vi "SMU_IV dual.vi"() -> ()   [LabVIEW 2022 SP3]
uses:
  <vilib>/Analysis/1siggen.llb/Ramp Pattern by Delta.vi
  Agilent U2722/Public/Configure/Configure Channel (Current).vi
  Agilent U2722/Public/Configure/Configure Channel (Voltage).vi
  Agilent U2722/Public/Data/Read Output (Single).vi
  <vilib>/Utility/file.llb/Write Delimited Spreadsheet (DBL).vi
  Agilent U2722/Agilent U2722.lvlib
  <vilib>/Analysis/NI_AALBase.lvlib
panel:
  in  "Tab Control":enum32{"Device Setup"}(tab)
  in  "Voltage Range 2":u16(ring) items=["2 Volts", "20 Volts"]
  in  "Current Range 2":u16(ring)=4 items=["1 uA", "10 uA", "100 uA", "1 mA", "10 mA", "120 mA"]
  in  "Current Limit  2":dbl=0.005 format="%#_2p"
  in  "Voltage Range":u16(ring) items=["2 Volts", "20 Volts"]
  in  "Starting Voltage (V)":dbl
  in  "Stopping Voltage (V)":dbl=1.0
  in  "Voltage Interval  (DV)":dbl format="%#_2g"
  in  "Current Range":u16(ring)=4 items=["1 uA", "10 uA", "100 uA", "1 mA", "10 mA", "120 mA"]
  in  "VISA resource name":refnum<visa-resource-name>
  in  "Drain - Source Channel":u16(ring)=1 items=["Channel 1"=1, "Channel 2"=2, "Channel 3"=3]
  in  "PLC":i32
  in  "Current Limit":dbl=0.005 format="%#_2p"
  in  "Interval Time (s)":dbl=1.0 caption="Delay Time (s)"
  in  "Starting Voltage (V) 2":dbl
  in  "Stopping Voltage (V) 2":dbl=1.0
  in  "Voltage Interval 2 (DV)":dbl format="%#_2g"
  in  "Gate - Source Channel":u16(ring)=2 items=["Channel 1"=1, "Channel 2"=2, "Channel 3"=3]
  in  "output file path":path
  out "XY Graph":cluster{"Y":dbl[], "Y":dbl[]}[](graph)
  out "XY Graph 2":cluster{"Y":dbl[], "Y":dbl[]}[](graph)
  out "XY Graph 4":cluster{"Y":dbl[], "Y":dbl[]}[](graph)
  out "XY Graph 3":cluster{"Y":dbl[], "Y":dbl[]}[](graph)
  in  "VISA resource name 2":refnum<visa-resource-name>
  in  "Voltage Range 3":u16(ring) items=["2 Volts", "20 Volts"]
  in  "Starting Voltage (V) 3":dbl
  in  "Stopping Voltage (V) 3":dbl=1.0
  in  "Voltage Interval  (DV) 2":dbl format="%#_2g"
  in  "Current Range 3":u16(ring)=4 items=["1 uA", "10 uA", "100 uA", "1 mA", "10 mA", "120 mA"]
  in  "Drain - Source Channel  2":u16(ring)=1 items=["Channel 1"=1, "Channel 2"=2, "Channel 3"=3]
  in  "PLC 2":i32
  in  "Current Limit  4":dbl=0.005 format="%#_2p"
  in  "Interval Time (s) 2":dbl=1.0 caption="Delay Time (s)"
  in  "Starting Voltage (V) 4":dbl
  in  "Stopping Voltage (V) 4":dbl=1.0
  in  "Voltage Interval 2 (DV)\n 2":dbl format="%#_2g"
  in  "Gate - Source Channel  2":u16(ring)=2 items=["Channel 1"=1, "Channel 2"=2, "Channel 3"=3]
  in  "output file path 2":path
  in  "Current Limit  3":dbl=0.005 format="%#_2p"
  in  "Current Range 4":u16(ring)=4 items=["1 uA", "10 uA", "100 uA", "1 mA", "10 mA", "120 mA"]
  in  "Voltage Range 2":u16(ring) items=["2 Volts", "20 Volts"]
  # "Drain Source Voltage Setting"
  # "Gate Source Voltage Setting"
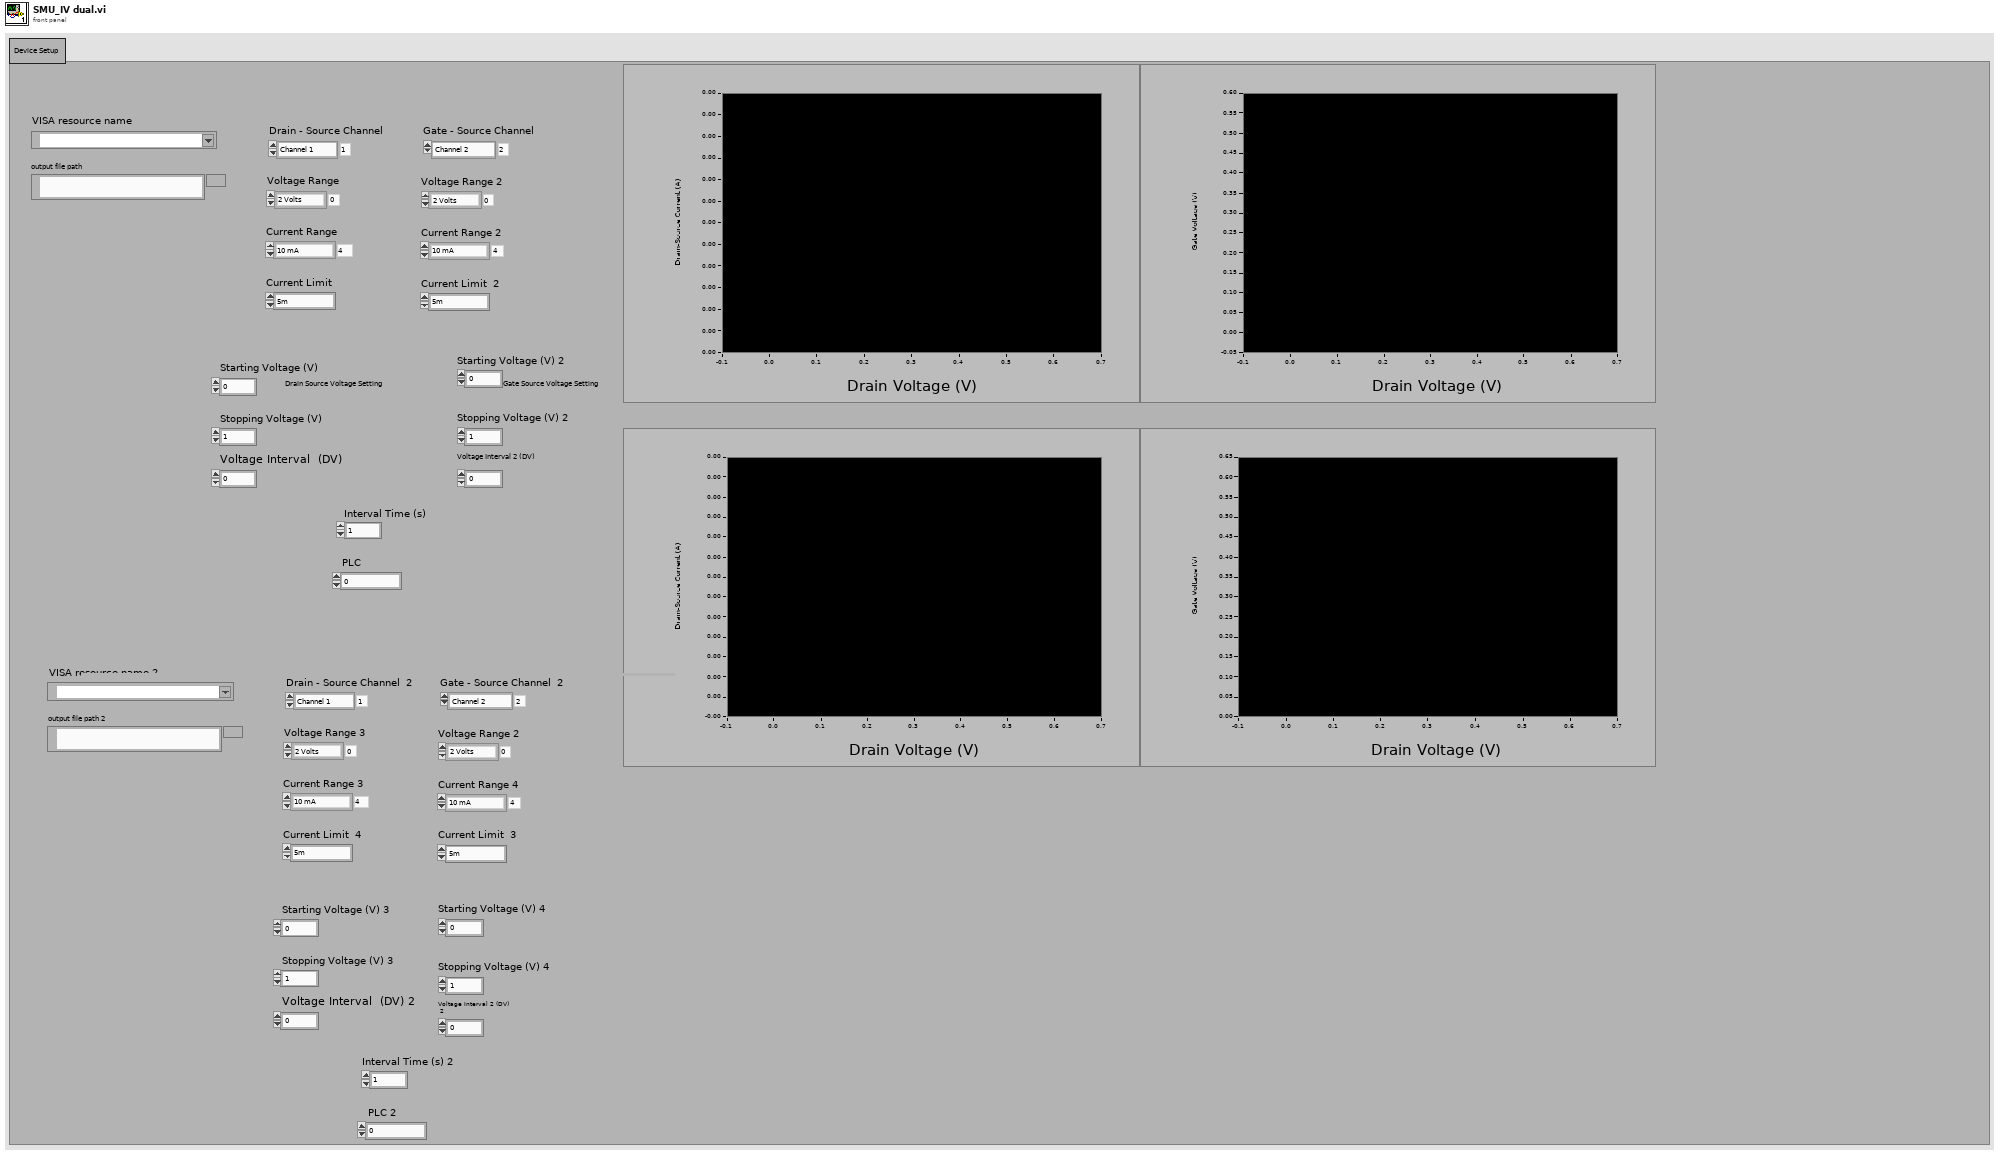
[diagram p1: front panel]
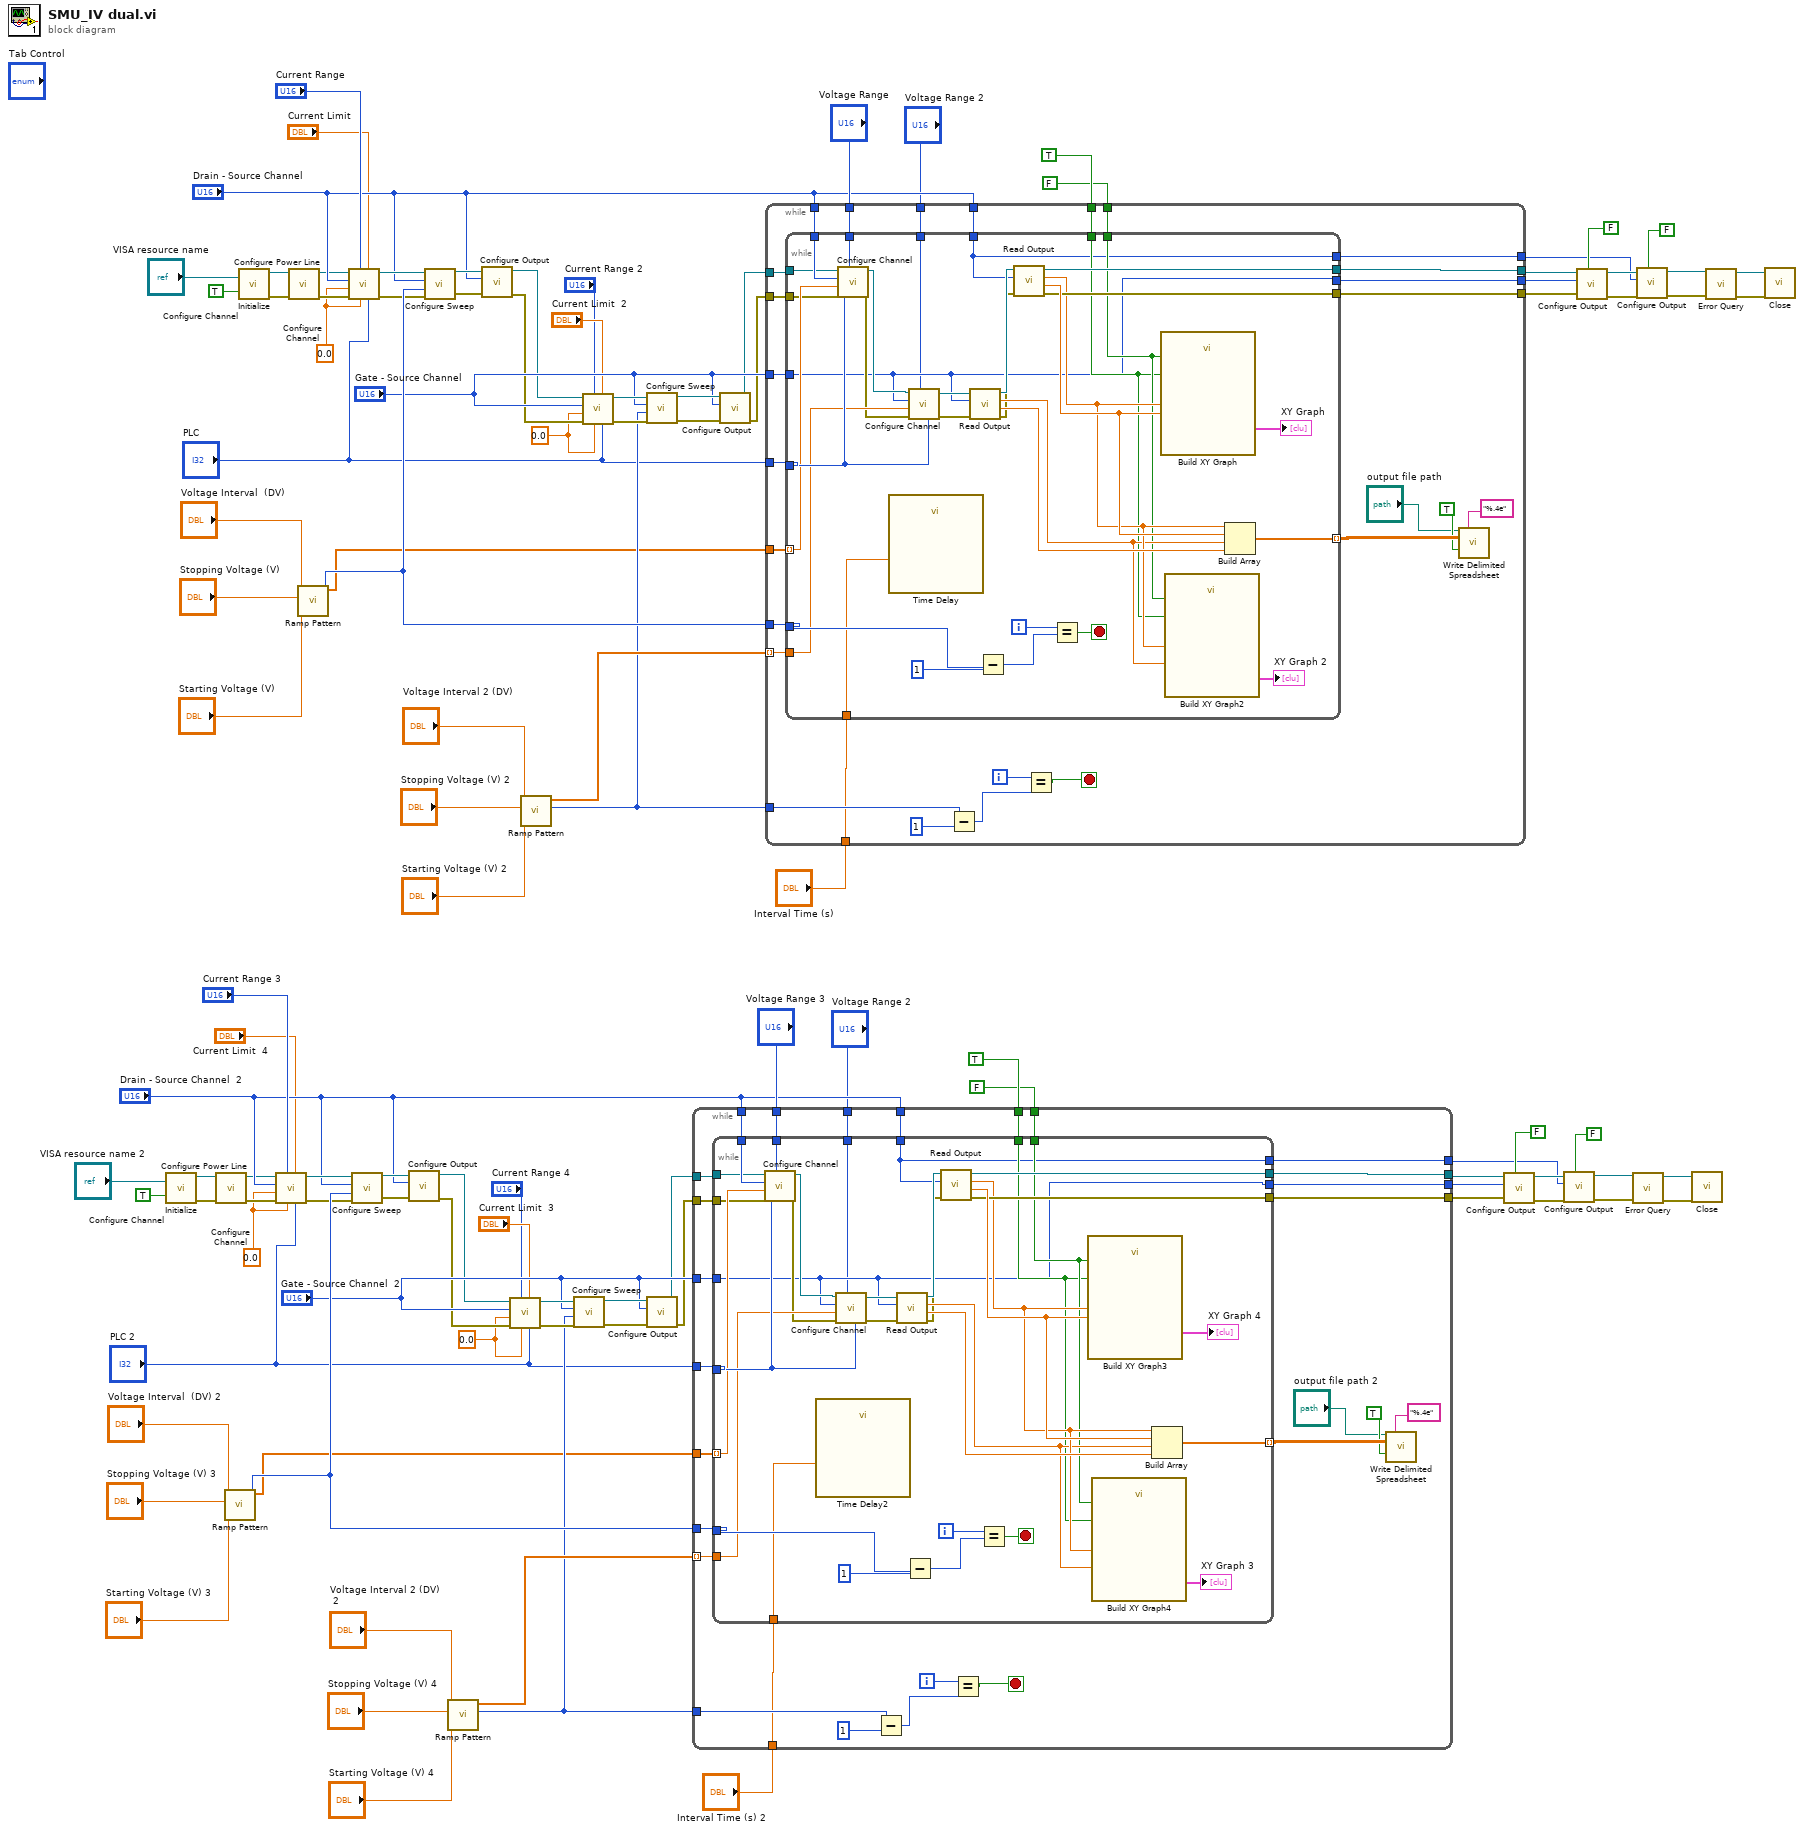
[diagram p0: block diagram]
diagram:
  w3 = 0.0
  w2 = 0.0
  w57 = 0.0
  w56 = 0.0
  n1 = call "Initialize.vi"("ID Query (True)"=TRUE, "VISA resource name"="VISA resource name 2") -> ("error out"=w49:errorcluster, "VISA resource name out"=w48:refnum<visa-resource-name>)  [unwired: 8 in]
  n2 = call "Configure Power Line.vi"("error in (no error)"=w49, "VISA resource name"=w48) -> ("error out"=w32:errorcluster, "VISA resource name out"=w19:refnum<visa-resource-name>)  [unwired: 8 in]
  n3 = call-poly <vilib>:"Ramp Pattern.vi"("start"="Starting Voltage (V) 3", "end"="Stopping Voltage (V) 3", "delta"="Voltage Interval  (DV) 2") -> ("samples"=w39:i32, "Ramp Pattern"=w22:dbl[])  [unwired: 6 in, 1 out]
  n4 = call "Initialize.vi"("ID Query (True)"=TRUE, "VISA resource name"="VISA resource name") -> ("error out"=w103:errorcluster, "VISA resource name out"=w102:refnum<visa-resource-name>)  [unwired: 8 in]
  n5 = call-poly "Configure Channel.vi"("Power Line Cycles (0)"="PLC 2", "Current Limit (1.0 uA)"="Current Limit  4", "Triggered Level (1.0 mA)"=w2, "Current Range (0: 1 uA)"="Current Range 3", "error in (no error)"=w32, "Output Level (1.0 mA)"=w2, "Channel (1: Channel 1)"="Drain - Source Channel  2", "VISA resource name"=w19) -> ("error out"=w36:errorcluster, "VISA resource name out"=w37:refnum<visa-resource-name>)  [unwired: 2 in]
  n6 = call "Configure Power Line.vi"("error in (no error)"=w103, "VISA resource name"=w102) -> ("error out"=w86:errorcluster, "VISA resource name out"=w73:refnum<visa-resource-name>)  [unwired: 8 in]
  n7 = call-poly <vilib>:"Ramp Pattern.vi"("start"="Starting Voltage (V)", "end"="Stopping Voltage (V)", "delta"="Voltage Interval  (DV)") -> ("samples"=w93:i32, "Ramp Pattern"=w76:dbl[])  [unwired: 6 in, 1 out]
  n8 = call-poly "Configure Channel.vi"("Power Line Cycles (0)"="PLC", "Current Limit (1.0 uA)"="Current Limit", "Triggered Level (1.0 mA)"=w56, "Current Range (0: 1 uA)"="Current Range", "error in (no error)"=w86, "Output Level (1.0 mA)"=w56, "Channel (1: Channel 1)"="Drain - Source Channel", "VISA resource name"=w73) -> ("error out"=w90:errorcluster, "VISA resource name out"=w91:refnum<visa-resource-name>)  [unwired: 2 in]
  n9 = call "Configure Sweep.vi"("error in (no error)"=w36, "Sweep Points (1)"=w39, "Channel (1: Channel 1)"="Drain - Source Channel  2", "VISA resource name"=w37) -> ("error out"=w40:errorcluster, "VISA resource name out"=w41:refnum<visa-resource-name>)  [unwired: 6 in]
  n10 = call "Configure Output.vi"("error in (no error)"=w40, "Channel (1: Channel 1)"="Drain - Source Channel  2", "VISA resource name"=w41) -> ("error out"=w17:errorcluster, "VISA resource name out"=w18:refnum<visa-resource-name>)  [unwired: 7 in]
  n11 = call "Configure Sweep.vi"("error in (no error)"=w90, "Sweep Points (1)"=w93, "Channel (1: Channel 1)"="Drain - Source Channel", "VISA resource name"=w91) -> ("error out"=w94:errorcluster, "VISA resource name out"=w95:refnum<visa-resource-name>)  [unwired: 6 in]
  n12 = call-poly <vilib>:"Ramp Pattern.vi"("start"="Starting Voltage (V) 4", "end"="Stopping Voltage (V) 4", "delta"="Voltage Interval 2 (DV)\n 2") -> ("samples"=w25:i32, "Ramp Pattern"=w26:dbl[])  [unwired: 6 in, 1 out]
  n13 = call "Configure Output.vi"("error in (no error)"=w94, "Channel (1: Channel 1)"="Drain - Source Channel", "VISA resource name"=w95) -> ("error out"=w71:errorcluster, "VISA resource name out"=w72:refnum<visa-resource-name>)  [unwired: 7 in]
  n14 = call-poly "Configure Channel.vi"("Power Line Cycles (0)"="PLC 2", "Current Limit (1.0 uA)"="Current Limit  3", "Triggered Level (1.0 mA)"=w3, "Current Range (0: 1 uA)"="Current Range 4", "error in (no error)"=w17, "Output Level (1.0 mA)"=w3, "Channel (1: Channel 1)"="Gate - Source Channel  2", "VISA resource name"=w18) -> ("error out"=w31:errorcluster, "VISA resource name out"=w30:refnum<visa-resource-name>)  [unwired: 2 in]
  n15 = call-poly <vilib>:"Ramp Pattern.vi"("start"="Starting Voltage (V) 2", "end"="Stopping Voltage (V) 2", "delta"="Voltage Interval 2 (DV)") -> ("samples"=w79:i32, "Ramp Pattern"=w80:dbl[])  [unwired: 6 in, 1 out]
  n16 = call "Configure Sweep.vi"("error in (no error)"=w31, "Sweep Points (1)"=w25, "Channel (1: Channel 1)"="Gate - Source Channel  2", "VISA resource name"=w30) -> ("error out"=w28:errorcluster, "VISA resource name out"=w29:refnum<visa-resource-name>)  [unwired: 6 in]
  n17 = call-poly "Configure Channel.vi"("Power Line Cycles (0)"="PLC", "Current Limit (1.0 uA)"="Current Limit  2", "Triggered Level (1.0 mA)"=w57, "Current Range (0: 1 uA)"="Current Range 2", "error in (no error)"=w71, "Output Level (1.0 mA)"=w57, "Channel (1: Channel 1)"="Gate - Source Channel", "VISA resource name"=w72) -> ("error out"=w85:errorcluster, "VISA resource name out"=w84:refnum<visa-resource-name>)  [unwired: 2 in]
  n18 = call "Configure Sweep.vi"("error in (no error)"=w85, "Sweep Points (1)"=w79, "Channel (1: Channel 1)"="Gate - Source Channel", "VISA resource name"=w84) -> ("error out"=w82:errorcluster, "VISA resource name out"=w83:refnum<visa-resource-name>)  [unwired: 6 in]
  n19 = call "Configure Output.vi"("error in (no error)"=w28, "Channel (1: Channel 1)"="Gate - Source Channel  2", "VISA resource name"=w29) -> ("error out"=w16:errorcluster, "VISA resource name out"=w15:refnum<visa-resource-name>)  [unwired: 7 in]
  n20 = while {
    tunnel: TRUE -> [w135]
    tunnel: FALSE -> [w134]
    tunnel: "PLC 2" -> [w133]
    tunnel: "Interval Time (s) 2" -> [w118]
    tunnel: w39 -> [w132]
    tunnel: "Voltage Range 3" -> [w131]
    tunnel: "Gate - Source Channel  2" -> [w130]
    tunnel: w26 -> [w129] mode=indexing
    tunnel: w25 -> [w125]
    tunnel: [w123] -> w24
    tunnel: [w122] -> w23
    tunnel: w22 -> [w121]
    tunnel: "Drain - Source Channel  2" -> [w120]
    tunnel: "Drain - Source Channel  2" -> [w119]
    tunnel: w16 -> [w110]
    tunnel: w15 -> [w117]
    tunnel: [w112] -> w9
    tunnel: [w111] -> w8
    tunnel: "Voltage Range 2" -> [w109]
    i -> [w127]
    stop <- w126 stop-if-true
    n21 = while {
      tunnel: w132 -> [w165]
      tunnel: w118 -> [w164]
      tunnel: w133 -> [w160]
      tunnel: w135 -> [w141]
      tunnel: w134 -> [w142]
      tunnel: [w149] -> w123
      tunnel: [w162] -> w122
      tunnel: w130 -> [w140]
      tunnel: w131 -> [w137]
      tunnel: w129 -> [w159]
      tunnel: [w152] -> w115 mode=indexing
      tunnel: w121 -> [w151] mode=indexing
      tunnel: w120 -> [w150]
      tunnel: w119 -> [w139]
      tunnel: w117 -> [w146]
      tunnel: [w140] -> w112
      tunnel: [w139] -> w111
      tunnel: w110 -> [w138]
      tunnel: w109 -> [w136]
      i -> [w161]
      stop <- w163 stop-if-true
      n22 = call-poly "Configure Channel.vi"("Power Line Cycles (0)"=w160, "Voltage Range (0: 2 Volts)"=w137, "error in (no error)"=w138, "Output Level (1.0 V)"=w151, "Channel (1: Channel 1)"=w150, "VISA resource name"=w146) -> ("error out"=w144:errorcluster, "VISA resource name out"=w145:refnum<visa-resource-name>)  [unwired: 4 in]
      n23 = call "Time Delay2"("Delay Time (s)"=w164) -> ()  [unwired: 10 in, 1 out]
      n24 = call-poly "Configure Channel.vi"("Power Line Cycles (0)"=w160, "Voltage Range (0: 2 Volts)"=w136, "error in (no error)"=w144, "Output Level (1.0 V)"=w159, "Channel (1: Channel 1)"=w140, "VISA resource name"=w145) -> ("error out"=w157:errorcluster, "VISA resource name out"=w158:refnum<visa-resource-name>)  [unwired: 4 in]
      n25 = call-poly "Read Output.vi"("error in (no error)"=w157, "Channel (1: Channel 1)"=w140, "VISA resource name"=w158) -> ("error out"=w143:errorcluster, "Actual Current Level (A)"=w156:dbl, "Actual Voltage Level (V)"=w148:dbl, "VISA resource name out"=w147:refnum<visa-resource-name>)  [unwired: 5 in]
      n26 = Subtract(x=w165, y=1 ("x")) -> (x-y=w167:i32)
      n27 = call-poly "Read Output.vi"("error in (no error)"=w143, "Channel (1: Channel 1)"=w139, "VISA resource name"=w147) -> ("error out"=w162:errorcluster, "Actual Current Level (A)"=w166:dbl, "Actual Voltage Level (V)"=w154:dbl, "VISA resource name out"=w149:refnum<visa-resource-name>)  [unwired: 5 in]
      n28 = Equal?(x=w161, y=w167) -> (x = y?=w163:bool)
      n29 = call "Build XY Graph3"("Enable"=w141, "Reset"=w142, "Y Input"=w166, "X Input"=w154) -> ("XY Graph"=→"XY Graph 4":cluster{"X":dbl[], "Y":dbl[]}[])  [unwired: 6 in, 1 out]
      n30 = call "Build XY Graph4"("Enable"=w141, "Reset"=w142, "Y Input"=w148, "X Input"=w154) -> ("XY Graph"=→"XY Graph 3":cluster{"X":dbl[], "Y":dbl[]}[])  [unwired: 6 in, 1 out]
      n31 = Build Array(w154, w166, w148, w156) -> (w152:dbl[])
    }
    n32 = Subtract(x=w125, y=1 ("x")) -> (x-y=w124:i32)
    n33 = Equal?(x=w127, y=w124) -> (x = y?=w126:bool)
    n34 = call-poly <vilib>:"Write Delimited Spreadsheet.vi"("file path (dialog if empty)"="output file path 2", "format (%.3f)"="%.4e", "2D data"=w115, "append to file? (new file:F)"=TRUE) -> ()  [unwired: 10 in, 2 out]
  }
  n35 = call "Configure Output.vi"("error in (no error)"=w82, "Channel (1: Channel 1)"="Gate - Source Channel", "VISA resource name"=w83) -> ("error out"=w70:errorcluster, "VISA resource name out"=w69:refnum<visa-resource-name>)  [unwired: 7 in]
  n36 = while {
    tunnel: TRUE -> [w195]
    tunnel: FALSE -> [w194]
    tunnel: "PLC" -> [w193]
    tunnel: "Interval Time (s)" -> [w178]
    tunnel: w93 -> [w192]
    tunnel: "Voltage Range" -> [w191]
    tunnel: "Gate - Source Channel" -> [w190]
    tunnel: w80 -> [w189] mode=indexing
    tunnel: w79 -> [w185]
    tunnel: [w183] -> w78
    tunnel: [w182] -> w77
    tunnel: w76 -> [w181]
    tunnel: "Drain - Source Channel" -> [w180]
    tunnel: "Drain - Source Channel" -> [w179]
    tunnel: w70 -> [w170]
    tunnel: w69 -> [w177]
    tunnel: [w172] -> w63
    tunnel: [w171] -> w62
    tunnel: "Voltage Range 2" -> [w169]
    i -> [w187]
    stop <- w186 stop-if-true
    n37 = while {
      tunnel: w192 -> [w225]
      tunnel: w178 -> [w224]
      tunnel: w193 -> [w220]
      tunnel: w195 -> [w201]
      tunnel: w194 -> [w202]
      tunnel: [w209] -> w183
      tunnel: [w222] -> w182
      tunnel: w190 -> [w200]
      tunnel: w191 -> [w197]
      tunnel: w189 -> [w219]
      tunnel: [w212] -> w175 mode=indexing
      tunnel: w181 -> [w211] mode=indexing
      tunnel: w180 -> [w210]
      tunnel: w179 -> [w199]
      tunnel: w177 -> [w206]
      tunnel: [w200] -> w172
      tunnel: [w199] -> w171
      tunnel: w170 -> [w198]
      tunnel: w169 -> [w196]
      i -> [w221]
      stop <- w223 stop-if-true
      n38 = call-poly "Configure Channel.vi"("Power Line Cycles (0)"=w220, "Voltage Range (0: 2 Volts)"=w197, "error in (no error)"=w198, "Output Level (1.0 V)"=w211, "Channel (1: Channel 1)"=w210, "VISA resource name"=w206) -> ("error out"=w204:errorcluster, "VISA resource name out"=w205:refnum<visa-resource-name>)  [unwired: 4 in]
      n39 = call "Time Delay"("Delay Time (s)"=w224) -> ()  [unwired: 10 in, 1 out]
      n40 = call-poly "Configure Channel.vi"("Power Line Cycles (0)"=w220, "Voltage Range (0: 2 Volts)"=w196, "error in (no error)"=w204, "Output Level (1.0 V)"=w219, "Channel (1: Channel 1)"=w200, "VISA resource name"=w205) -> ("error out"=w217:errorcluster, "VISA resource name out"=w218:refnum<visa-resource-name>)  [unwired: 4 in]
      n41 = call-poly "Read Output.vi"("error in (no error)"=w217, "Channel (1: Channel 1)"=w200, "VISA resource name"=w218) -> ("error out"=w203:errorcluster, "Actual Current Level (A)"=w216:dbl, "Actual Voltage Level (V)"=w208:dbl, "VISA resource name out"=w207:refnum<visa-resource-name>)  [unwired: 5 in]
      n42 = Subtract(x=w225, y=1 ("x")) -> (x-y=w227:i32)
      n43 = call-poly "Read Output.vi"("error in (no error)"=w203, "Channel (1: Channel 1)"=w199, "VISA resource name"=w207) -> ("error out"=w222:errorcluster, "Actual Current Level (A)"=w226:dbl, "Actual Voltage Level (V)"=w214:dbl, "VISA resource name out"=w209:refnum<visa-resource-name>)  [unwired: 5 in]
      n44 = Equal?(x=w221, y=w227) -> (x = y?=w223:bool)
      n45 = call "Build XY Graph"("Enable"=w201, "Reset"=w202, "Y Input"=w226, "X Input"=w214) -> ("XY Graph"=→"XY Graph":cluster{"X":dbl[], "Y":dbl[]}[])  [unwired: 6 in, 1 out]
      n46 = call "Build XY Graph2"("Enable"=w201, "Reset"=w202, "Y Input"=w208, "X Input"=w214) -> ("XY Graph"=→"XY Graph 2":cluster{"X":dbl[], "Y":dbl[]}[])  [unwired: 6 in, 1 out]
      n47 = Build Array(w214, w226, w208, w216) -> (w212:dbl[])
    }
    n48 = Subtract(x=w185, y=1 ("x")) -> (x-y=w184:i32)
    n49 = Equal?(x=w187, y=w184) -> (x = y?=w186:bool)
    n50 = call-poly <vilib>:"Write Delimited Spreadsheet.vi"("file path (dialog if empty)"="output file path", "format (%.3f)"="%.4e", "2D data"=w175, "append to file? (new file:F)"=TRUE) -> ()  [unwired: 10 in, 2 out]
  }
  n51 = call "Configure Output.vi"("Enable Output (T: Enable)"=FALSE, "error in (no error)"=w23, "Channel (1: Channel 1)"=w9, "VISA resource name"=w24) -> ("error out"=w12:errorcluster, "VISA resource name out"=w14:refnum<visa-resource-name>)  [unwired: 6 in]
  n52 = call "Configure Output.vi"("Enable Output (T: Enable)"=FALSE, "error in (no error)"=w12, "Channel (1: Channel 1)"=w8, "VISA resource name"=w14) -> ("error out"=w11:errorcluster, "VISA resource name out"=w13:refnum<visa-resource-name>)  [unwired: 6 in]
  n53 = call "Configure Output.vi"("Enable Output (T: Enable)"=FALSE, "error in (no error)"=w77, "Channel (1: Channel 1)"=w63, "VISA resource name"=w78) -> ("error out"=w66:errorcluster, "VISA resource name out"=w68:refnum<visa-resource-name>)  [unwired: 6 in]
  n54 = call "Error Query.vi"("error in (no error)"=w11, "VISA resource name"=w13) -> ("error out"=w43:errorcluster, "VISA resource name out"=w42:refnum<visa-resource-name>)  [unwired: 6 in, 2 out]
  n55 = call "Configure Output.vi"("Enable Output (T: Enable)"=FALSE, "error in (no error)"=w66, "Channel (1: Channel 1)"=w62, "VISA resource name"=w68) -> ("error out"=w65:errorcluster, "VISA resource name out"=w67:refnum<visa-resource-name>)  [unwired: 6 in]
  n56 = call "Close.vi"("error in (no error)"=w43, "VISA resource name"=w42) -> ()  [unwired: 9 in, 1 out]
  n57 = call "Error Query.vi"("error in (no error)"=w65, "VISA resource name"=w67) -> ("error out"=w97:errorcluster, "VISA resource name out"=w96:refnum<visa-resource-name>)  [unwired: 6 in, 2 out]
  n58 = call "Close.vi"("error in (no error)"=w97, "VISA resource name"=w96) -> ()  [unwired: 9 in, 1 out]
